vi "Intensity Graph to Image.vi"(7 "Gray?":bool, 8 "error in":errorcluster, 10 "image":dbl[][](array[numeric]), 11 "Intensity Graph Refnum":refnum<vi>) -> (0 "error out":errorcluster, 3 "Image Out":T1)   [LabVIEW 2023]
uses:
  <vilib>/vision/Image Controls.llb/IMAQ Image.ctl
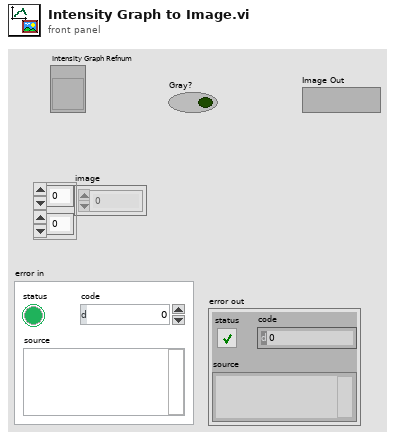
[diagram p1: front panel]
types:
  T1 = typedef "IMAQ Image.ctl" = refnum<image>
  T2 = typedef "Image Type" = u32
  T3 = typedef "imagedata.ctl" = cluster{"image type":i32, "image depth":i32, "image":u8[], "mask":u8[], "colors":u32[], "Rectangle":cluster{"left":i16, "top":i16, "right":i16, "bottom":i16}}
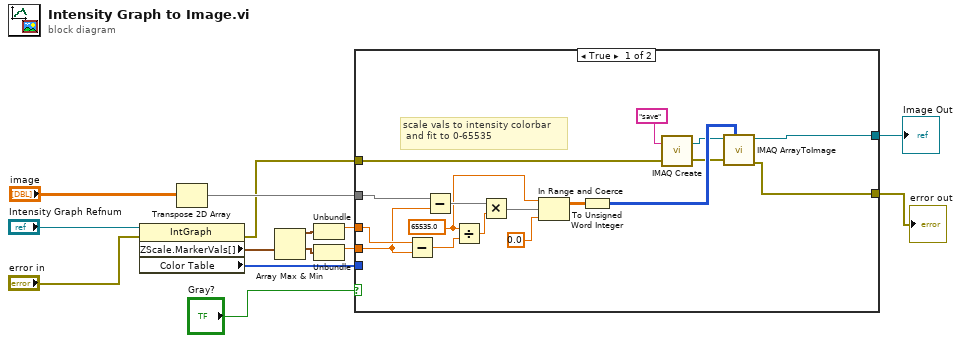
[diagram p0: block diagram]
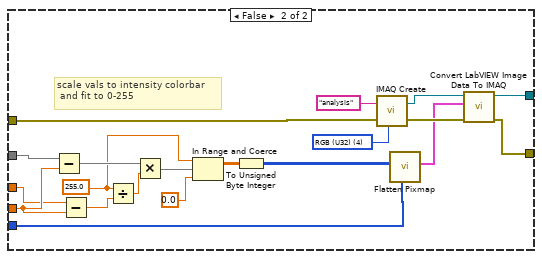
[diagram p2: hidden frame]
diagram:
  n1 = property class="IntGraph"(reference="Intensity Graph Refnum", error in="error in") -> (error out=w9:errorcluster, "ZScale.MarkerVals[]"=w12:cluster{dbl, u32}[], "Color Table"=w11:u32[])  [unwired: 1 out]
  n2 = Transpose 2D Array(2D array="image") -> (transposed array=w10:dbl[][])
  n3 = Array Max & Min(array=w12) -> (max value=w4:cluster{dbl, u32}, min value=w3:cluster{dbl, u32})  [unwired: 2 out]
  n4 = Unbundle(w4) -> (w1:dbl)  [unwired: 1 out]
  n5 = Unbundle(w3) -> (w2:dbl)  [unwired: 1 out]
  n6 = case shown="True" "Gray?" {
    tunnel: w11 -> [_ w44]
    tunnel: w10 -> [w23 w42]
    tunnel: w9 -> [w22 w41]
    tunnel: [w21 w40] -> w8
    tunnel: [w20 w39] -> w7
    tunnel: w2 -> [w18 w38]
    tunnel: w1 -> [w19 w37]
    frame True {
      w27 = 65535.0
      # "scale vals to intensity colorbar\n and fit to 0-65535"
      n7 = Subtract(x=w19, y=w18) -> (x-y=w30:dbl)
      n8 = Subtract(x=w23, y=w18) -> (x-y=w31:dbl[][])
      n9 = Divide(x=w27, y=w30) -> (x/y=w29:dbl)
      n10 = Multiply(x=w31, y=w29) -> (x*y=w26:dbl[][])
      n11 = In Range and Coerce(upper limit=w27, x=w26, lower limit=0.0) -> (coerced(x)=w25:dbl[][])  [unwired: 1 out]
      n12 = To Unsigned Word Integer(number=w25) -> (unsigned 16bit integer=w24:u16[][])
      n13 = call "IMAQ Create"("Image Name"="save", "error in (no error)"=w22) -> ("New Image"=w16:T1, "error out"=w17:errorcluster)  [unwired: 3 in]
      n14 = call "IMAQ ArrayToImage"("Image Pixels (U16)"=w24, "error in (no error)"=w17, "Image"=w16) -> ("error out"=w21:errorcluster, "Image Out"=w20:T1)  [unwired: 7 in]
    }
    frame False {
      w35 = T2 4 items=["Grayscale (U8)", "Grayscale (I16)", "Grayscale (SGL)", "Complex (CSG)", "RGB (U32)", "HSL (U32)", "RGB (U64)", "Grayscale (U16)"] ("Image Type")
      w47 = 255.0
      # "scale vals to intensity colorbar\n and fit to 0-255"
      n15 = Subtract(x=w42, y=w38) -> (x-y=w51:dbl[][])
      n16 = Subtract(x=w37, y=w38) -> (x-y=w50:dbl)
      n17 = Divide(x=w47, y=w50) -> (x/y=w49:dbl)
      n18 = Multiply(x=w51, y=w49) -> (x*y=w46:dbl[][])
      n19 = In Range and Coerce(upper limit=w47, x=w46, lower limit=0.0) -> (coerced(x)=w45:dbl[][])  [unwired: 1 out]
      n20 = To Unsigned Byte Integer(number=w45) -> (unsigned 8bit integer=w43:u8[][])
      n21 = call "IMAQ Create"("Image Name"="analysis", "Image Type"=w35, "error in (no error)"=w41) -> ("New Image"=w32:T1, "error out"=w34:errorcluster)  [unwired: 2 in]
      n22 = call <vilib>:"Flatten Pixmap.vi"("colors"=w44, "8-bit pixmap"=w43) -> ("image data"=w33:T3)  [unwired: 9 in]
      n23 = call "Convert LabVIEW Image Data To IMAQ.vi"("error in (no error)"=w34, "Image Data"=w33, "Image In"=w32) -> ("error out"=w40:errorcluster, "Image Out"=w39:T1)  [unwired: 7 in]
    }
  }
  "error out" <- w8
  "Image Out" <- w7
